vi "Send and receive test 1.vi"() -> ()   [LabVIEW 2012]
uses:
  <vilib>/Utility/inputDevices.llb/closeKeyboard.vi
  <vilib>/Utility/inputDevices.llb/keyboardAcquire.vi
panel:
  out "count":i32
  in  "ESTOP":bool
  in  "Step Size":i32=5
  in  "PC Status":i32=1
  in  "Pan Camera":i32(slide)=1500 scale=500.0..2500.0
  out "Motors Speed":i32(knob) scale=500.0..2500.0
  out "Rudders Direction":i32(knob) scale=500.0..2500.0
  in  "Balance motors":i32(slide) scale=-200.0..200.0
  out "Starboard\nMotor":i32
  out "Port\nMotor":i32
  in  "Balance Rudders":i32(slide) scale=-200.0..200.0
  out "Right\nRubber":i32
  out "Left\nRudder":i32
  out "byte array":u8[](array[numeric]) format="%02x"
  out "String Received":string
  out "return count":u32
  out "bytes written":u32
  out "Blinky":bool
  in  "String":string="$CS1500P1500R1500L1500P1500H   1\n"
  in  "stop":bool
  in  "VISA resource name":refnum<visa-resource-name>="COM6"
  # "USE THE ARROW KEYS TO CHANGE THE MOTOR SPEED AND RUDDER POSITION"
  # "DRAG THE SLIDERS TO BALANCE THE MOTOR SPEEDS, BALANCE THE RUDDER ANGLES AND PAN THE CAMERA."
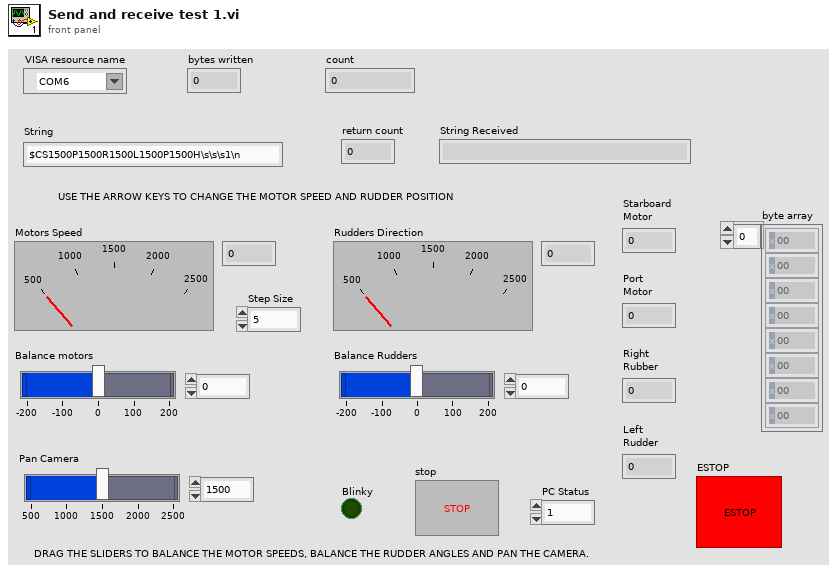
[diagram p1: front panel]
types:
  T1 = enum16{"0", "1", "2", "3", "4", "5", "6", "7", "8", "9", "A", "B", "C", "D", "E", "F", "G", "H", "I", "J", "K", "L", "M", "N", "O", "P", "Q", "R", "S", "T", "U", "V", "W", "X", "Y", "Z", "F1", "F2", "F3", "F4", "F5", "F6", "F7", "F8", "F9", "F10", "F11", "F12", "F13", "F14", "F15", "ADD", "BACK", "BACKSLASH", "CAPITAL", "COMMA", "DECIMAL", "DELETE", "DIVIDE", "DOWN", "END", "EQUALS", "ESCAPE", "GRAVE (`)", "HOME", "INSERT", "LBRACKET", "LCONTROL", "LEFT", "L ALT", "LSHIFT", "LWIN", "MINUS", "MULTIPLY", "NEXT", "NUMLOCK", "NUMPAD_0", "NUMPAD_1", "NUMPAD_2", "NUMPAD_3", "NUMPAD_4", "NUMPAD_5", "NUMPAD_6", "NUMPAD_7", "NUMPAD_8", "NUMPAD_9", "PAUSE", "PERIOD", "PRIOR (PG UP)", "RBRACKET", "RCONTROL", "RETURN", "RIGHT", "R ALT", "RSHIFT", "RWIN", "SCROLL", "SEMICOLON", "SLASH", "SPACE", "SUBTRACT", "TAB", "UP", "ENTER (num pad)", "' (quote)"}[]
  T2 = enum16{"0", "1", "2", "3", "4", "5", "6", "7", "8", "9", "A", "B", "C", "D", "E", "F", "G", "H", "I", "J", "K", "L", "M", "N", "O", "P", "Q", "R", "S", "T", "U", "V", "W", "X", "Y", "Z", "F1", "F2", "F3", "F4", "F5", "F6", "F7", "F8", "F9", "F10", "F11", "F12", "F13", "F14", "F15", "ADD", "BACK", "BACKSLASH", "CAPITAL", "COMMA", "DECIMAL", "DELETE", "DIVIDE", "DOWN", "END", "EQUALS", "ESCAPE", "GRAVE (`)", "HOME", "INSERT", "LBRACKET", "LCONTROL", "LEFT", "L ALT", "LSHIFT", "LWIN", "MINUS", "MULTIPLY", "NEXT", "NUMLOCK", "NUMPAD_0", "NUMPAD_1", "NUMPAD_2", "NUMPAD_3", "NUMPAD_4", "NUMPAD_5", "NUMPAD_6", "NUMPAD_7", "NUMPAD_8", "NUMPAD_9", "PAUSE", "PERIOD", "PRIOR (PG UP)", "RBRACKET", "RCONTROL", "RETURN", "RIGHT", "R ALT", "RSHIFT", "RWIN", "SCROLL", "SEMICOLON", "SLASH", "SPACE", "SUBTRACT", "TAB", "UP", "ENTER (num pad)", "' (quote)"}
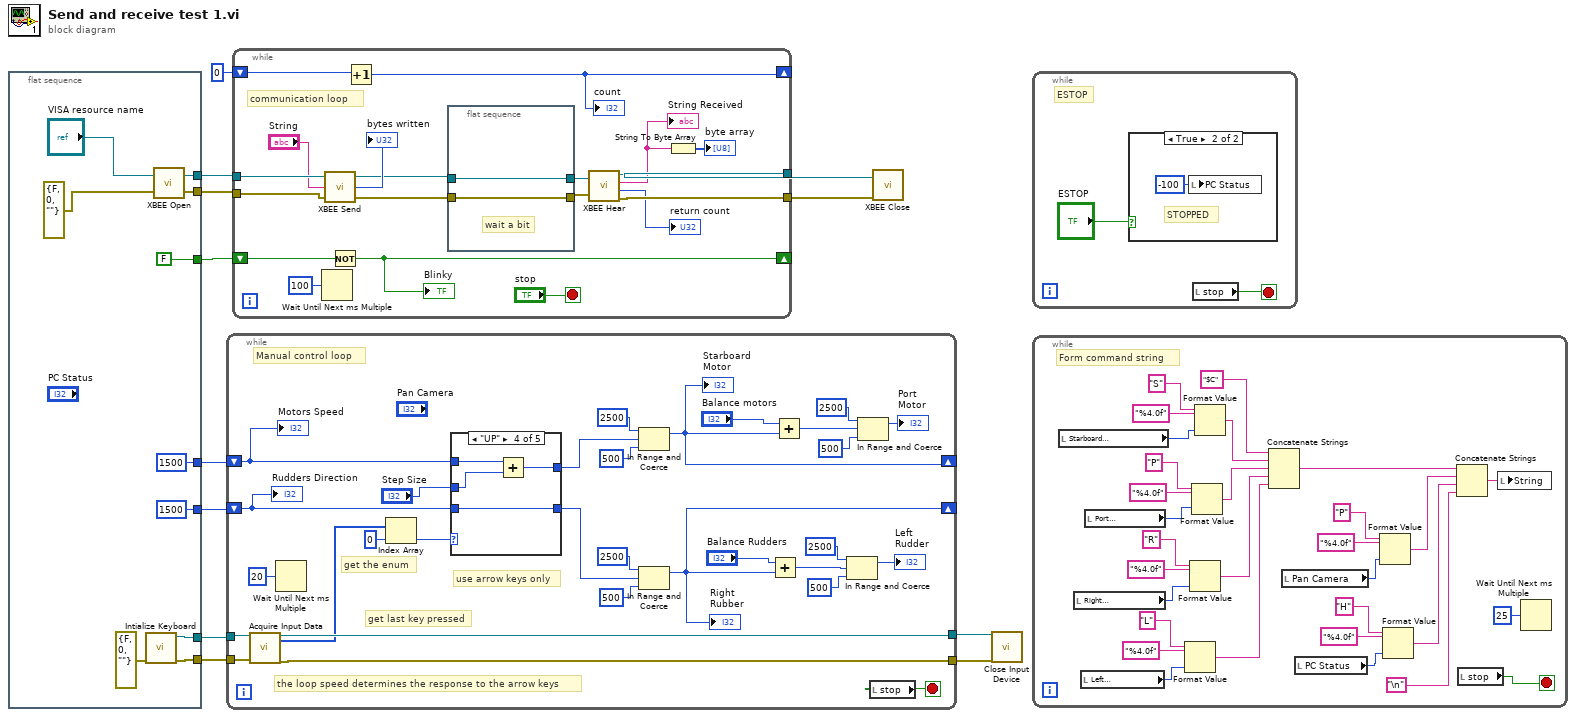
[diagram p0: block diagram]
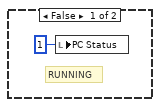
[diagram p2: hidden frame]
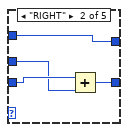
[diagram p4: hidden frame]
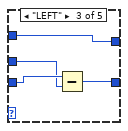
[diagram p5: hidden frame]
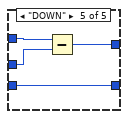
[diagram p6: hidden frame]
diagram:
  n1 = flat-sequence {
    tunnel: [w22] -> w12
    tunnel: [w21] -> w11
    tunnel: [FALSE] -> w8
    tunnel: [w19] -> w7
    tunnel: [w17] -> w6
    tunnel: [1500] -> w3
    tunnel: [1500] -> w2
    frame #0 {
      n2 = call <vilib>:"Intialize Keyboard.vi"("error in (no error)"=errorcluster {"status"=FALSE, "code"=0, "source"=""}) -> ("error out"=w19:errorcluster, "device ID"=w17:refnum<k1>)  [unwired: 9 in]
      n3 = call "XBEE Open.vi"("error in"=errorcluster {"status"=FALSE, "code"=0, "source"=""}, "VISA resource name"="VISA resource name") -> ("error out"=w21:errorcluster, "VISA resource name out"=w22:refnum<visa-resource-name>)
    }
  }
  n4 = while {
    tunnel: w7 -> [w52]
    tunnel: w6 -> [w51]
    tunnel: [w50] -> w5
    tunnel: [w49] -> w4
    shift-right: [w35] -> _
    shift-left: w2 -> [w44]
    shift-right: [w33] -> _
    shift-left: w3 -> [w43]
    stop <- w24 stop-if-true
    # "use arrow keys only"
    # "Manual control loop"
    # "get the enum"
    # "the loop speed determines the response to the arrow keys"
    # "get last key pressed"
    n5 = call-poly <vilib>:"Acquire Input Data.vi"("device ID"=w51, "error in (no error)"=w52) -> ("device ID"=w49:refnum<k1>, "keys pressed"=w48:T1, "error out"=w50:errorcluster)  [unwired: 15 in]
    n6 = Wait Until Next ms Multiple(millisecond multiple=u32 20) -> ()  [unwired: 1 out]
    n7 = Index Array(array=w48, index=0) -> (element=w46:T2)
    n8 = case shown="\"UP\"" w46 {
      tunnel: w44 -> [w54 w58 w62 w64 w68]
      tunnel: [w54 w58 w62 w65 w69] -> w42
      tunnel: w43 -> [w53 w57 w60 w66 w70]
      tunnel: [w53 w56 w61 w66 w70] -> w37
      tunnel: "Step Size" -> [_ w55 w59 w63 w67]
      frame "0", Default {
      }
      frame "RIGHT" {
        n9 = Add(x=w57, y=w55) -> (x+y=w56:i32)
      }
      frame "LEFT" {
        n10 = Subtract(x=w60, y=w59) -> (x-y=w61:i32)
      }
      frame "UP" {
        n11 = Add(x=w64, y=w63) -> (x+y=w65:i32)
      }
      frame "DOWN" {
        n12 = Subtract(x=w68, y=w67) -> (x-y=w69:i32)
      }
    }
    n13 = In Range and Coerce(upper limit=2500, x=w42, lower limit=500) -> (coerced(x)=w35:i32)  [unwired: 1 out]
    "Starboard\nMotor" <- w35
    n14 = In Range and Coerce(upper limit=2500, x=w37, lower limit=500) -> (coerced(x)=w33:i32)  [unwired: 1 out]
    "Right\nRubber" <- w33
    n15 = Add(x="Balance Rudders", y=w33) -> (x+y=w26:i32)
    n16 = Add(x="Balance motors", y=w35) -> (x+y=w30:i32)
    n17 = In Range and Coerce(upper limit=2500, x=w26, lower limit=500) -> (coerced(x)=→"Left\nRudder":i32)  [unwired: 1 out]
    n18 = In Range and Coerce(upper limit=2500, x=w30, lower limit=500) -> (coerced(x)=→"Port\nMotor":i32)  [unwired: 1 out]
    n19 = local read "stop"() -> (w24:bool)
    "Motors Speed" <- w44
    "Rudders Direction" <- w43
  }
  n20 = while {
    tunnel: w12 -> [w88]
    tunnel: w11 -> [w87]
    tunnel: [w82] -> w10
    tunnel: [w81] -> w9
    shift-right: [w85] -> _
    shift-left: w8 -> [w86]
    shift-right: [w71] -> _
    shift-left: 0 -> [w72]
    stop <- "stop" stop-if-true
    # "communication loop"
    n21 = Wait Until Next ms Multiple(millisecond multiple=u32 100) -> ()  [unwired: 1 out]
    n22 = call "XBEE Send.vi"("error in (no error)"=w87, "String"="String", "VISA resource name"=w88) -> ("error out"=w76:errorcluster, "return count"=→"bytes written":u32, "VISA resource name out"=w77:refnum<visa-resource-name>)
    n23 = Not(x=w86) -> (.not. x?=w85:bool)
    "Blinky" <- w85
    n24 = Increment(x=w72) -> (x+1=w71:i32)
    "count" <- w71
    n25 = flat-sequence {
      tunnel: w77 -> [w91]
      tunnel: w76 -> [w90]
      tunnel: [w91] -> w75
      tunnel: [w90] -> w74
      frame #0 {
        # "wait a bit"
      }
    }
    n26 = call "XBEE Hear.vi"("VISA resource name"=w75, "error in (no error)"=w74) -> ("VISA resource name out"=w82:refnum<visa-resource-name>, "String Received"=w79:string, "return count"=→"return count":u32, "error out"=w81:errorcluster)
    "String Received" <- w79
    n27 = String To Byte Array(string=w79) -> (unsigned byte array=→"byte array":u8[])
  }
  n28 = call "XBEE Close.vi"("error in (no error)"=w9, "VISA resource name"=w10) -> ()
  n29 = call-poly <vilib>:"Close Input Device.vi"("error in (no error)"=w5, "device ID"=w4) -> ()  [unwired: 8 in, 1 out]
  n30 = while {
    stop <- w93 stop-if-true
    # "ESTOP"
    n31 = case shown="True" "ESTOP" {
      frame False {
        # "RUNNING"
        n32 = local write "PC Status"(1 ("PC Status")) -> ()
      }
      frame True {
        # "STOPPED"
        n33 = local write "PC Status"(-100) -> ()
      }
    }
    n34 = local read "stop"() -> (w93:bool)
  }
  n35 = while {
    stop <- w125 stop-if-true
    # "Form command string"
    n36 = local read "Starboard\nMotor"() -> (w122:i32)
    n37 = local read "Right\nRubber"() -> (w113:i32)
    n38 = local read "Left\nRudder"() -> (w110:i32)
    n39 = local read "Port\nMotor"() -> (w119:i32)
    n40 = Format Value(string ("")="L", format string="%4.0f", value (0)=w110) -> (output string=w108:string)
    n41 = Format Value(string ("")="R", format string="%4.0f", value (0)=w113) -> (output string=w109:string)
    n42 = Format Value(string ("")="P", format string="%4.0f", value (0)=w119) -> (output string=w116:string)
    n43 = Format Value(string ("")="S", format string="%4.0f", value (0)=w122) -> (output string=w117:string)
    n44 = Concatenate Strings("$C", w117, w116, w109, w108) -> (w100:string)
    n45 = local read "Pan Camera"() -> (w104:i32)
    n46 = local read "PC Status"() -> (w101:i32)
    n47 = Format Value(string ("")="P", format string="%4.0f", value (0)=w104) -> (output string=w99:string)
    n48 = Format Value(string ("")="H", format string="%4.0f", value (0)=w101) -> (output string=w98:string)
    n49 = Concatenate Strings(w100, w99, w98, "\n") -> (w105:string)
    n50 = local read "stop"() -> (w125:bool)
    n51 = local write "String"(w105) -> ()
    n52 = Wait Until Next ms Multiple(millisecond multiple=u32 25) -> ()  [unwired: 1 out]
  }
